vi "manip_status_loop.vi"(8 "error in":errorcluster, 11 "I2C interface":T3) -> (0 "error out":errorcluster)   [LabVIEW 2013]
uses:
  i2c_interface.ctl
  fpga_reference.ctl
  status_filter.ctl
  Common/i2c_status.ctl
  <vilib>/Platform/TimedLoop/XDataNode/timing_clust.ctl
  <vilib>/Platform/TimedLoop/XDataNode/nitl_modes.ctl
  <vilib>/Platform/TimedLoop/XDataNode/wakeup.ctl
  <vilib>/Platform/TimedLoop/XDataNode/XDataNode.xnode
  <vilib>/Platform/TimedLoop/XDataNode/XDNodeRunTimeDep.lvlib
panel:
  out "Dt statistics":cluster{"Min":u16, "Max":u16, "Mean":sgl}
  in  "Show before":i32=3
  out "Above threshold":i32
  in  "Dt threshold":u16=500
  in  "Error len max":i32=2000
  in  "Update":bool
  out "Match count":i32
  in  "Display len":i32=16
  out "Filtered status":string
  in  "Filter >=":T1=enum."I2C error"
  in  "Reset":bool
  in  "Filter":T2={"Argument"=-1, "Code"=enum."Invalid", "Code >="=TRUE, "Bus"=-1}
  out "Status/sec":i32
  out "Num reports":i32
  out "Num status":i32
  out "Error log":string
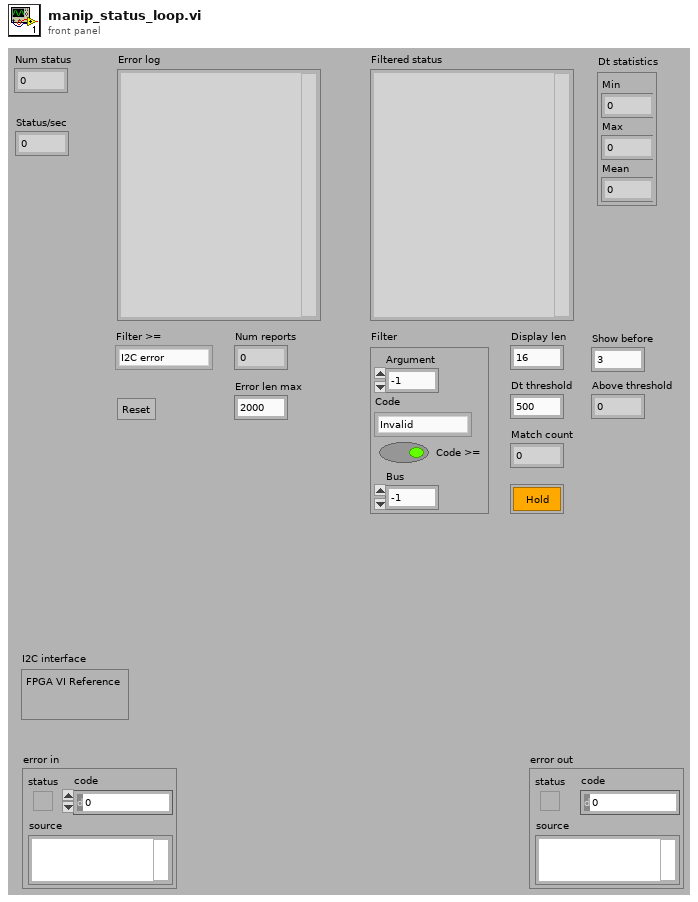
[diagram p1: front panel]
types:
  T1 = typedef "i2c_status.ctl" = enum8{"Invalid", "Command", "I2C start", "Trigger wait", "TX data wait", "Sequence", "Receive data", "I2C error", "Address NACK", "Data NACK", "SDA stuck", "SCL stuck", "Bad command"}
  T2 = typedef "status_filter.ctl" = cluster{"Argument":i16, "Code":T1, "Code >=":bool, "Bus":i16}
  T3 = typedef "i2c_interface.ctl" = cluster{"FPGA VI Reference":T4}
  T4 = typedef "fpga_reference.ctl" = refnum<k20>
  T5 = typedef "XDNodeRunTimeDep.lvlib/timing_clust.ctl" = cluster{"Expected End [f-1]":u64, "Actual End [f-1]":u64, "Finished Late? [f-1]":bool, "Expected End [i-1]":u64, "Actual End [i-1]":u64, "Finished Late? [i-1]":bool, "Expected Start [i]":u64, "Actual Start [i]":u64, "Expected Start [f]":u64, "Actual Start [f]":u64, "Source Name":string, "Structure Name":string, "Period":i64, "Deadline":i64, "Offset":i64, "Start":i64, "Priority":i32, "Timeout":i32, "Mode":T6, "Wakeup Reason":T7, "Error":errorcluster, "Source Type":string, "Secondary Source Type":string, "Global End Time":u64, "Global Start Time":u64, "Frame Duration":u64, "Iteration Duration":u64, "Assigned CPU":i32, "I/O Scan Engine Mode":u32}
  T6 = typedef "XDNodeRunTimeDep.lvlib/nitl_modes.ctl" = enum32{"No Change", "Process missed periods, maintain original phase", "Discard missed periods, maintain original phase", "Process missed periods, ignore original phase", "Discard missed periods, ignore original phase"}
  T7 = typedef "XDNodeRunTimeDep.lvlib/wakeup.ctl" = enum32{"Normal", "Aborted", "Asynchronous wakeup", "Timing source error", "Timed loop error", "Timeout"}
  T8 = typedef "i2c_status_cluster.ctl" = cluster{"Bus":u8, "Timestamp":u16, "Code":T1, "Argument":u8}
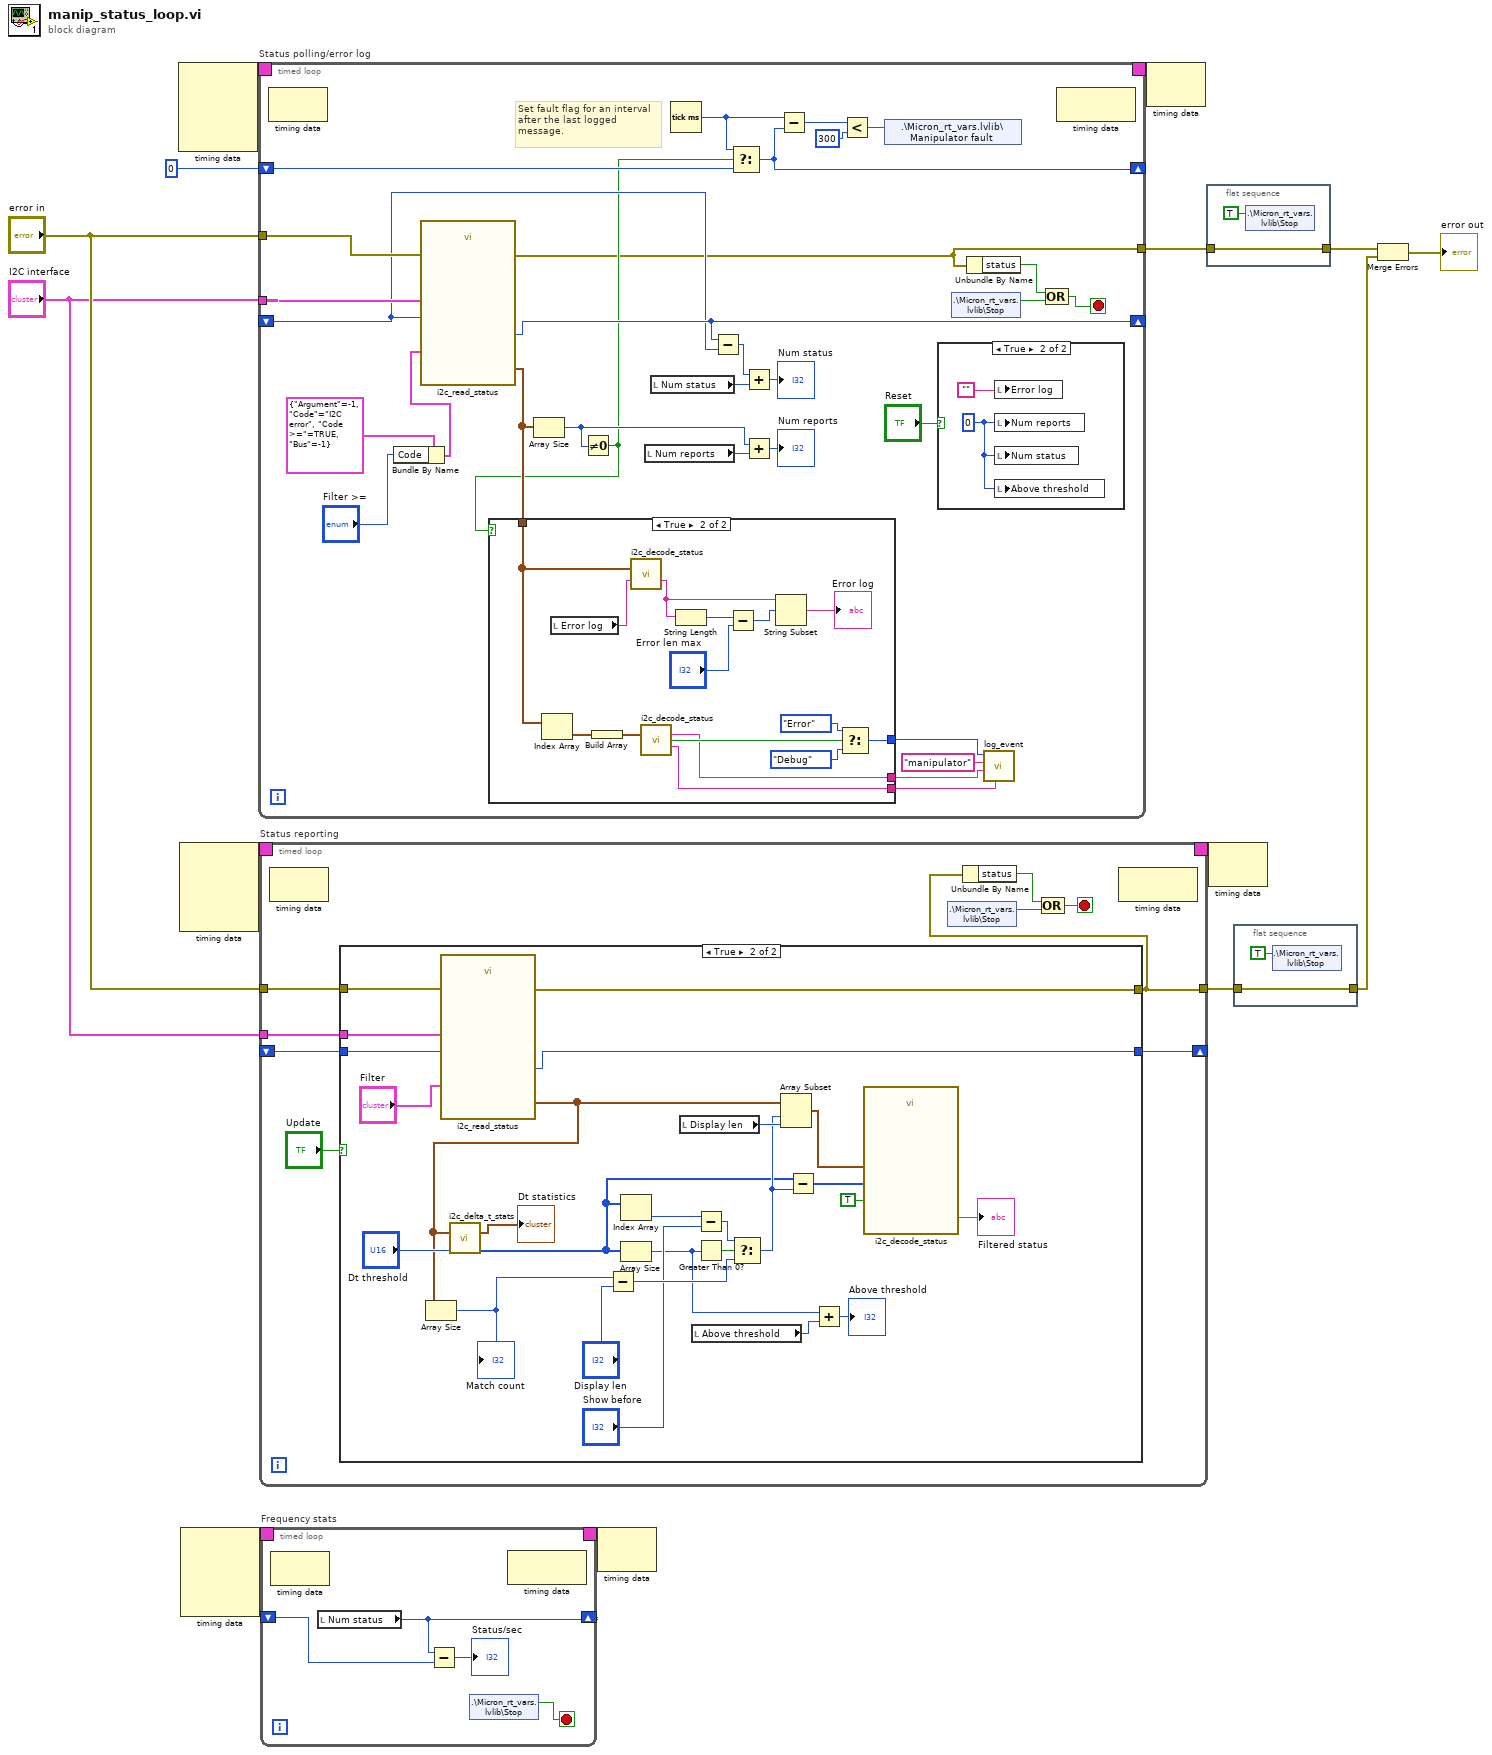
[diagram p0: block diagram]
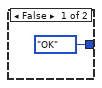
[diagram p4: hidden frame]
diagram:
  n1 = node-c288() -> (w10:T5)  [unwired: 4 in]
  n2 = node-c288() -> (w4:T5)  [unwired: 4 in]
  n3 = node-c288() -> (w12:T5)  [unwired: 4 in]
  n4 = timed-loop "Status polling/error log" {
    tunnel: "error in" -> [w34]
    tunnel: "I2C interface" -> [w44]
    tunnel: [w19] -> w13
    shift-right: [w39] -> _
    shift-left: u32 0 ("millisecond timer value") -> [w40]
    shift-right: [w28] -> _
    shift-left: _ -> [w27]
    timing: w10 -> [_]
    timing-out: [_] -> w9
    stop <- w41 stop-if-true
    # "Set fault flag for an interval\nafter the last logged\nmessage."
    n5 = node-c288() -> ()  [unwired: 1 in, 1 out]
    n6 = Bundle By Name(cluster=T2 {"Argument"=-1, "Code"=enum."I2C error", "Code >="=TRUE, "Bus"=-1} ("Filter"), "Code"="Filter >=") -> (w21:T2)
    n7 = call "i2c_read_status.vi"("I2C interface"=w44, "Start index"=w27, "Filter"=w21, "error in"=w34) -> ("End index"=w28:i32, "Result"=w25:T8[], "error out"=w19:errorcluster)  [unwired: 13 in]
    n8 = Array Size(array=w25) -> (size(s)=w26:i32)
    n9 = Not Equal To 0?(x=w26) -> (x != 0?=w24:bool)
    n10 = case shown="True" w24 {
      tunnel: w25 -> [_ w58]
      tunnel: [enum16{"OK", "Debug", "Warn", "Error"}."OK" ("Severity") w54] -> w15
      tunnel: [_ w53] -> w17
      tunnel: [_ w52] -> w16
      frame False {
      }
      frame True {
        n11 = Index Array(array=w58) -> (element=w57:T8)  [unwired: 1 in]
        n12 = local read "Error log"() -> (w64:string)
        n13 = Build Array(w57) -> (w56:T8[])
        n14 = call "i2c_decode_status.vi"("Input"=w58, "Initial string"=w64) -> ("Result"=w60:string)  [unwired: 11 in, 2 out]
        n15 = call "i2c_decode_status.vi"("Input"=w56) -> ("Last code string"=w53:string, "Last error"=w55:bool, "Result"=w52:string)  [unwired: 12 in]
        n16 = String Length(string=w60) -> (length=w63:i32)
        n17 = Subtract(x=w63, y="Error len max") -> (x-y=w59:i32)
        n18 = String Subset(string=w60, offset (0)=w59) -> (substring=→"Error log":string)  [unwired: 1 in]
        n19 = Select(t=enum16{"OK", "Debug", "Warn", "Error"}."Error" ("Severity"), s=w55, f=enum16{"OK", "Debug", "Warn", "Error"}."Debug" ("Severity")) -> (s? t:f=w54:enum16{"OK", "Debug", "Warn", "Error"})
      }
    }
    n20 = local read "Num reports"() -> (w32:i32)
    n21 = local read "Num status"() -> (w31:i32)
    n22 = Tick Count (ms)() -> (millisecond timer value=w38:u32)
    n23 = Subtract(x=w28, y=w27) -> (x-y=w29:i32)
    n24 = Select(t=w38, s=w24, f=w40) -> (s? t:f=w39:u32)
    n25 = Add(x=w29, y=w31) -> (x+y=→"Num status":i32)
    n26 = Add(x=w26, y=w32) -> (x+y=→"Num reports":i32)
    n27 = Subtract(x=w38, y=w39) -> (x-y=w37:u32)
    n28 = Less?(x=w37, y=u32 300) -> (x < y?=w35:bool)
    n29 = shared-variable ".\\Micron_rt_vars.lvlib\\Manipulator fault"(w35) -> ()  [unwired: 1 in, 1 out]
    n30 = case shown="True" "Reset" {
      frame False {
      }
      frame True {
        w45 = 0 ("Num status")
        n31 = local write "Error log"("") -> ()
        n32 = local write "Num reports"(w45) -> ()
        n33 = local write "Num status"(w45) -> ()
        n34 = local write "Above threshold"(w45) -> ()
      }
    }
    n35 = shared-variable ".\\Micron_rt_vars.lvlib\\Stop"() -> (w42:bool)  [unwired: 2 out]
    n36 = Unbundle By Name(w19) -> ("status"=w43:bool)
    n37 = call "log_event.vi"("Message"=w16, "State"=w17, "Facility"="manipulator", "Severity"=w15) -> ()  [unwired: 7 in, 1 out]
    n38 = Compound Arithmetic op=OR(w43, w42) -> (w41:bool)
    n39 = node-c288() -> ()  [unwired: 1 in, 1 out]
  }
  n40 = timed-loop "Status reporting" {
    tunnel: "error in" -> [w69]
    tunnel: "I2C interface" -> [w73]
    tunnel: [w66] -> w2
    shift-right: [w68] -> _
    shift-left: _ -> [w67]
    timing: w4 -> [_]
    timing-out: [_] -> w3
    stop <- w70 stop-if-true
    n41 = node-c288() -> ()  [unwired: 1 in, 1 out]
    n42 = case shown="True" "Update" {
      tunnel: w73 -> [_ w101]
      tunnel: w69 -> [w74 w100]
      tunnel: [w75 w99] -> w68
      tunnel: w67 -> [w75 w98]
      tunnel: [w74 w92] -> w66
      frame False {
      }
      frame True {
        n43 = call "i2c_read_status.vi"("I2C interface"=w101, "Start index"=w98, "Filter"="Filter", "error in"=w100) -> ("End index"=w99:i32, "Result"=w85:T8[], "error out"=w92:errorcluster)  [unwired: 13 in]
        n44 = Array Size(array=w85) -> (size(s)=w94:i32)
        "Match count" <- w94
        n45 = call "i2c_delta_t_stats.vi"("Input"=w85, "Threshold"="Dt threshold") -> ("Results"=→"Dt statistics":cluster{"Min":u16, "Max":u16, "Mean":sgl}, "Big delta t"=w79:i32[])  [unwired: 12 in]
        n46 = Subtract(x=w94, y="Display len") -> (x-y=w86:i32)
        n47 = Index Array(array=w79) -> (element=w88:i32)  [unwired: 1 in]
        n48 = Array Size(array=w79) -> (size(s)=w77:i32)
        n49 = local read "Display len"() -> (w83:i32)
        n50 = local read "Above threshold"() -> (w76:i32)
        n51 = Subtract(x=w88, y="Show before") -> (x-y=w87:i32)
        n52 = Greater Than 0?(x=w77) -> (x > 0?=w89:bool)
        n53 = Select(t=w87, s=w89, f=w86) -> (s? t:f=w82:i32)
        n54 = Array Subset(array=w85, index=w82, length=w83) -> (w84:T8[])
        n55 = Subtract(x=w79, y=w82) -> (x-y=w81:i32[])
        n56 = Add(x=w77, y=w76) -> (x+y=→"Above threshold":i32)
        n57 = call "i2c_decode_status.vi"("Input"=w84, "Relative time"=TRUE, "Flag indices"=w81) -> ("Result"=→"Filtered status":string)  [unwired: 10 in, 2 out]
      }
    }
    n58 = shared-variable ".\\Micron_rt_vars.lvlib\\Stop"() -> (w71:bool)  [unwired: 2 out]
    n59 = Unbundle By Name(w66) -> ("status"=w72:bool)
    n60 = Compound Arithmetic op=OR(w72, w71) -> (w70:bool)
    n61 = node-c288() -> ()  [unwired: 1 in, 1 out]
  }
  n62 = timed-loop "Frequency stats" {
    timing: w12 -> [_]
    timing-out: [_] -> w11
    shift-right: [w107] -> _
    shift-left: _ -> [w106]
    stop <- w104 stop-if-true
    n63 = node-c288() -> ()  [unwired: 1 in, 1 out]
    n64 = local read "Num status"() -> (w107:i32)
    n65 = Subtract(x=w107, y=w106) -> (x-y=→"Status/sec":i32)
    n66 = shared-variable ".\\Micron_rt_vars.lvlib\\Stop"() -> (w104:bool)  [unwired: 2 out]
    n67 = node-c288() -> ()  [unwired: 1 in, 1 out]
  }
  n68 = node-c288(w11) -> ()  [unwired: 1 out]
  n69 = node-c288(w9) -> ()  [unwired: 1 out]
  n70 = flat-sequence {
    tunnel: w13 -> [w110]
    tunnel: [w110] -> w6
    frame #0 {
      n71 = shared-variable ".\\Micron_rt_vars.lvlib\\Stop"(TRUE ("Stop")) -> ()  [unwired: 2 out]
    }
  }
  n72 = node-c288(w3) -> ()  [unwired: 1 out]
  n73 = flat-sequence {
    tunnel: w2 -> [w112]
    tunnel: [w112] -> w1
    frame #0 {
      n74 = shared-variable ".\\Micron_rt_vars.lvlib\\Stop"(TRUE ("Stop")) -> ()  [unwired: 2 out]
    }
  }
  n75 = Merge Errors(w6, w1) -> (→"error out":errorcluster)
